vi "String.vi"() -> ()   [LabVIEW 2014]
panel:
  out "EOL Stations":string
  out "颜色代码":string
  in  "ST90 Error":T1
  in  "ST30 Error":T1
  in  "OPC.Var.ST30":T2
  in  "OPC.Var.ST90":T3
  in  "OPC.Var.PA50":T4
  in  "OPC.Var.PA30":T5
  in  "OPC.Var.PA10":T6
  in  "ST90打印测试":bool
  out "PA10托盘上载上限":dbl
  out "PA30托盘上载上限":dbl
  in  "ST30打印测试":bool
  out "2-nd Min":dbl
  out "1-st Max":dbl
  out "2-nd Max":dbl
  out "1-st Min":dbl
  out "客户代码":string
  out "产线编码":string
  out "供应商编码":string
  out "零件号":string
  out "物料代码":string
  out "项目类型":string
  in  "PA30托盘号":string
  in  "PA10托盘号":string
  in  "PA30料车号":string
  in  "PA10料车号":string
  in  "PA30数据库查询语句":string
  in  "PA10数据库查询语句":string
  out "来料信息":string
  out "PA30加工次数":dbl
  out "PA30最大光强":dbl
  out "PA30最小光强":dbl
  out "PA30工作速度":dbl
  out "PA30当前文件":string
  out "PA10加工次数":dbl
  out "PA10最大光强":dbl
  out "PA10最小光强":dbl
  out "PA10工作速度":dbl
  out "PA10当前文件":string
  out "ST90 扫描数据":string
  out "ST30 扫描数据":string
  out "PA60 扫描数据":string
  out "PA30 扫描数据":string
  out "PA20 扫描数据":string
  out "PA10 扫描数据":string
  out "PA50 扫描数据":string
  in  "数据库ID":string
  out "ST90 流水号":string
  out "ST30 流水号":string
  out "PA60 流水号":string
  out "PA50流水号":string
  out "PA30流水号":string
  out "PA20流水号":string
  out "PA10流水号":string
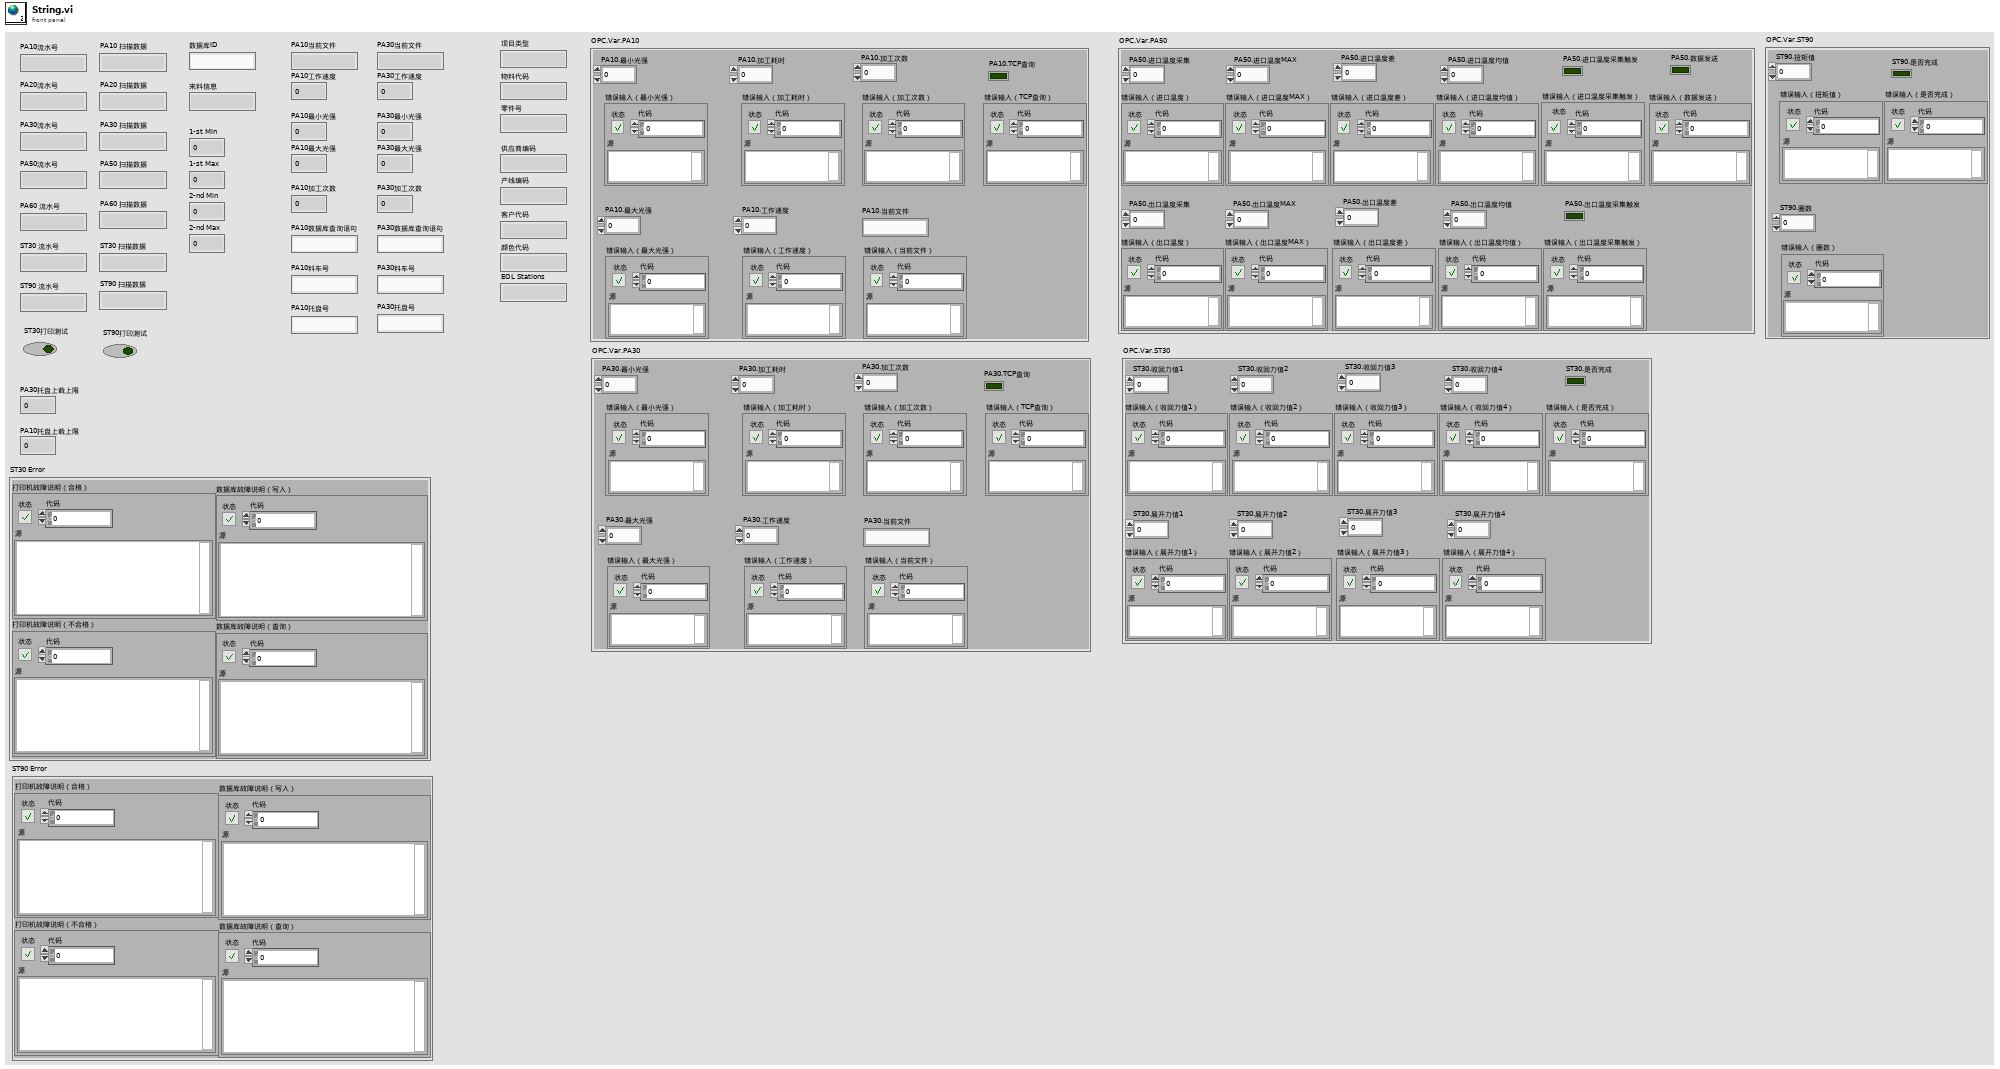
[diagram p1: front panel]
types:
  T1 = cluster{"打印机故障说明（合格）":errorcluster, "数据库故障说明（写入）":errorcluster, "打印机故障说明（不合格）":errorcluster, "数据库故障说明（查询）":errorcluster}
  T2 = cluster{"ST30.收回力值1":u16, "error in (no error)":errorcluster, "ST30.收回力值2":u16, "error in (no error) 3":errorcluster, "ST30.收回力值3":u16, "error in (no error) 5":errorcluster, "ST30.收回力值4":u16, "error in (no error) 7":errorcluster, "ST30.展开力值1":u16, "error in (no error) 2":errorcluster, "ST30.展开力值2":u16, "error in (no error) 4":errorcluster, "ST30.展开力值3":u16, "error in (no error) 6":errorcluster, "ST30.展开力值4":u16, "error in (no error) 9":errorcluster, "ST30.是否完成":bool, "error in (no error) 8":errorcluster}
  T3 = cluster{"ST90.扭矩值":u16, "error in (no error)":errorcluster, "ST90.圈数":u16, "error in (no error) 2":errorcluster, "ST90.是否完成":bool, "error in (no error) 7":errorcluster}
  T4 = cluster{"PA50.进口温度采集":u16, "error in (no error)":errorcluster, "PA50.进口温度MAX":u16, "error in (no error) 3":errorcluster, "PA50.进口温度差":u16, "error in (no error) 5":errorcluster, "PA50.进口温度均值":u16, "error in (no error) 7":errorcluster, "PA50.进口温度采集触发":bool, "error in (no error) 8":errorcluster, "PA50.出口温度采集":u16, "error in (no error) 2":errorcluster, "PA50.出口温度MAX":u16, "error in (no error) 4":errorcluster, "PA50.出口温度差":u16, "error in (no error) 6":errorcluster, "PA50.出口温度均值":u16, "error in (no error) 9":errorcluster, "PA50.出口温度采集触发":bool, "error in (no error) 10":errorcluster, "PA50.数据发送":bool, "error in (no error) 11":errorcluster}
  T5 = cluster{"PA30.最小光强":u16, "error in (no error)":errorcluster, "PA30.最大光强":u16, "error in (no error) 2":errorcluster, "PA30.加工耗时":u16, "error in (no error) 3":errorcluster, "PA30.工作速度":u16, "error in (no error) 4":errorcluster, "PA30.加工次数":u16, "error in (no error) 5":errorcluster, "PA30.当前文件":string, "error in (no error) 6":errorcluster, "PA30.TCP查询":bool, "error in (no error) 7":errorcluster}
  T6 = cluster{"PA10.最小光强":u16, "error in (no error)":errorcluster, "PA10.最大光强":u16, "error in (no error) 2":errorcluster, "PA10.加工耗时":u16, "error in (no error) 3":errorcluster, "PA10.工作速度":u16, "error in (no error) 4":errorcluster, "PA10.加工次数":u16, "error in (no error) 5":errorcluster, "PA10.当前文件":string, "error in (no error) 6":errorcluster, "PA10.TCP查询":bool, "error in (no error) 7":errorcluster}
diagram:
